vi "Forward For Inch.vi"(6 "error in (no error)":errorcluster, 8 "Angle":dbl, 9 "Speed":dbl, 10 "Distance":dbl, 11 "drive.lvclass":refnum<class "drive.lvclass">) -> (0 "error out":errorcluster, 3 "drive.lvclass":refnum<class "drive.lvclass">)   [LabVIEW 2015, in "drive.lvclass"]
uses:
  drive.lvclass
  drive.lvclass/drive.ctl
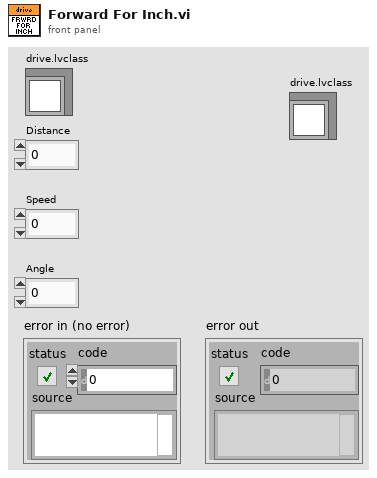
[diagram p1: front panel]
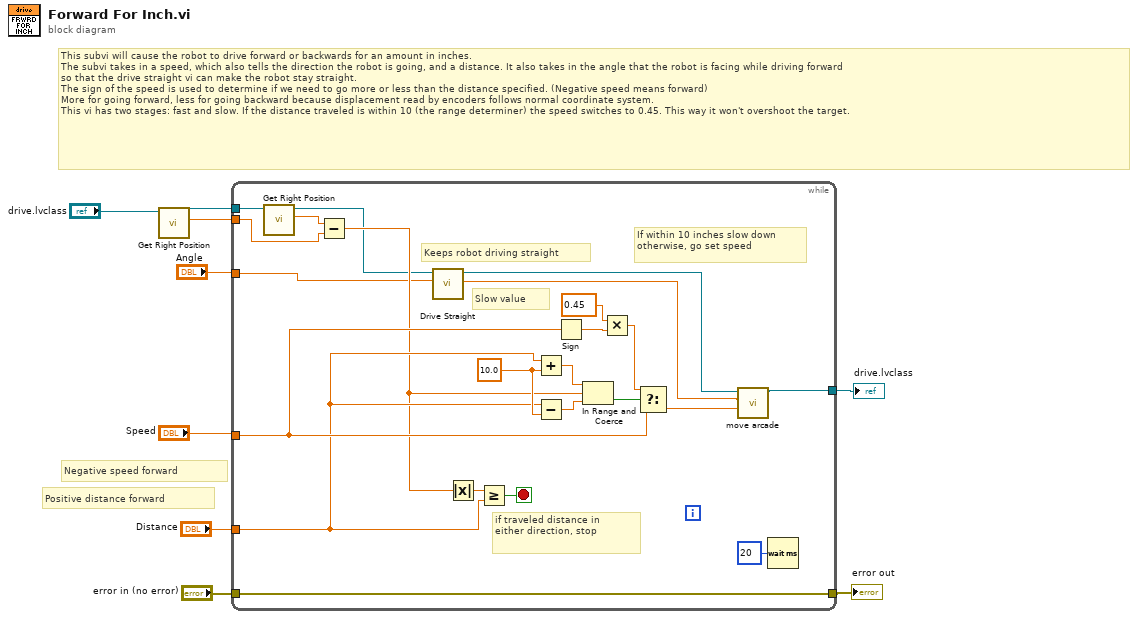
[diagram p0: block diagram]
diagram:
  # "Positive distance forward"
  # "Negative speed forward"
  # "This subvi will cause the robot to drive forward or backwards for an amount in inches.\nThe subvi takes in a speed, which also tells the direction the robot is going, and a distance. It also takes in the angle that the robot is facing while driving forward\nso that the drive straight vi can make the robot stay straight.\nThe sign of the speed is used to determine if we need to go more or less than the distance specified. (Negative speed means forward)\nMore for going forward, less for going backward because displacement read by encoders follows normal coordinate system. \nThis vi has two stages: fast and slow. If the distance traveled is within 10 (the range determiner) the speed switches to 0.45. This way it won't overshoot the target."
  n1 = call "Get Right Position.vi"("drive in"="drive.lvclass") -> ("RPosition"=w4:dbl, "drive out"=w3:refnum<class "drive.lvclass">)  [unwired: 9 in]
  n2 = while {
    tunnel: [w19] -> w6
    tunnel: "Distance" -> [w22]
    tunnel: "Speed" -> [w24]
    tunnel: "Angle" -> [w14]
    tunnel: w4 -> [w16]
    tunnel: w3 -> [w18]
    tunnel: "error in (no error)" -> [w10]
    tunnel: [w10] -> w1
    stop <- w21 stop-if-true
    w30 = 10.0
    # "if traveled distance in\neither direction, stop"
    # "If within 10 inches slow down\notherwise, go set speed"
    # "Keeps robot driving straight"
    # "Slow value"
    n3 = call "Get Right Position.vi"("drive in"=w18) -> ("RPosition"=w17:dbl, "drive out"=w12:refnum<class "drive.lvclass">)  [unwired: 9 in]
    n4 = Subtract(x=w17, y=w16) -> (x-y=w15:dbl)
    n5 = call "Drive Straight.vi"("Angle robot facing"=w14, "drive.lvclass"=w12) -> ("Arcade drive x"=w13:dbl, "drive.lvclass"=w11:refnum<class "drive.lvclass">)  [unwired: 8 in]
    n6 = Absolute Value(x=w15) -> (abs(x)=w23:dbl)
    n7 = Greater Or Equal?(x=w23, y=w22) -> (x >= y?=w21:bool)
    n8 = Add(x=w22, y=w30) -> (x+y=w28:dbl)
    n9 = Subtract(x=w22, y=w30) -> (x-y=w29:dbl)
    n10 = Sign(1:w24) -> (0:w26:dbl)
    n11 = In Range and Coerce(upper limit=w28, x=w15, lower limit=w29) -> (In Range?=w31:bool)  [unwired: 1 out]
    n12 = Multiply(x=0.45 ("t"), y=w26) -> (x*y=w25:dbl)
    n13 = Select(t=w25, s=w31, f=w24) -> (s? t:f=w20:dbl)
    n14 = call "move arcade.vi"("Forward Value"=w20, "Turn Value"=w13, "drive.lvclass"=w11) -> ("drive.lvclass"=w19:refnum<class "drive.lvclass">)  [unwired: 8 in]
    n15 = Wait (ms)(milliseconds to wait=u32 20) -> ()  [unwired: 1 out]
  }
  "drive.lvclass" <- w6
  "error out" <- w1
